vi "ErrorStructureDrawer-main.vi"(8 "Error In":errorcluster, 11 "VI reference":refnum<vi>) -> (0 "Error Out":errorcluster, 3 "VI reference (dup)":refnum<vi>)   [LabVIEW 2017, in "ErrorStructureDrawer.lvlib"]
doc: "Main VI for drawing an error structure around code using VI scripting."
uses:
  ErrorStructureDrawer.lvlib
panel:
  # "Copyright 2020, Stuart J. Box\n\nRedistribution and use in source and binary forms, with or without modification, are permitted provided that the following conditions are met:\n\n1. Redistributions of source code must retain the above copyright notice, this list of conditions and the following disclaimer.\n\n2. Redistributions in binary form must reproduce the above copyright notice, this list of conditions and the following disclaimer in the documentation and/or other materials provided with the distribution.\n\n3. Neither the name of the copyright holder nor the names of its contributors may be used to endorse or promote products derived from this software without specific prior written permission.\n\nTHIS SOFTWARE IS PROVIDED BY THE COPYRIGHT HOLDERS AND CONTRIBUTORS \"AS IS\" AND ANY EXPRESS OR IMPLIED WARRANTIES, INCLUDING, BUT NOT LIMITED TO, THE IMPLIED WARRANTIES OF MERCHANTABILITY AND FITNESS FOR A PARTICULAR PURPOSE ARE DISCLAIMED. IN NO EVENT SHALL THE COPYRIGHT HOLDER OR CONTRIBUTORS BE LIABLE FOR ANY DIRECT, INDIRECT, INCIDENTAL, SPECIAL, EXEMPLARY, OR CONSEQUENTIAL DAMAGES (INCLUDING, BUT NOT LIMITED TO, PROCUREMENT OF SUBSTITUTE GOODS OR SERVICES; LOSS OF USE, DATA, OR PROFITS; OR BUSINESS INTERRUPTION) HOWEVER CAUSED AND ON ANY THEORY OF LIABILITY, WHETHER IN CONTRACT, STRICT LIABILITY, OR TORT (INCLUDING NEGLIGENCE OR OTHERWISE) ARISING IN ANY WAY OUT OF THE USE OF THIS SOFTWARE, EVEN IF ADVISED OF THE POSSIBILITY OF SUCH DAMAGE."
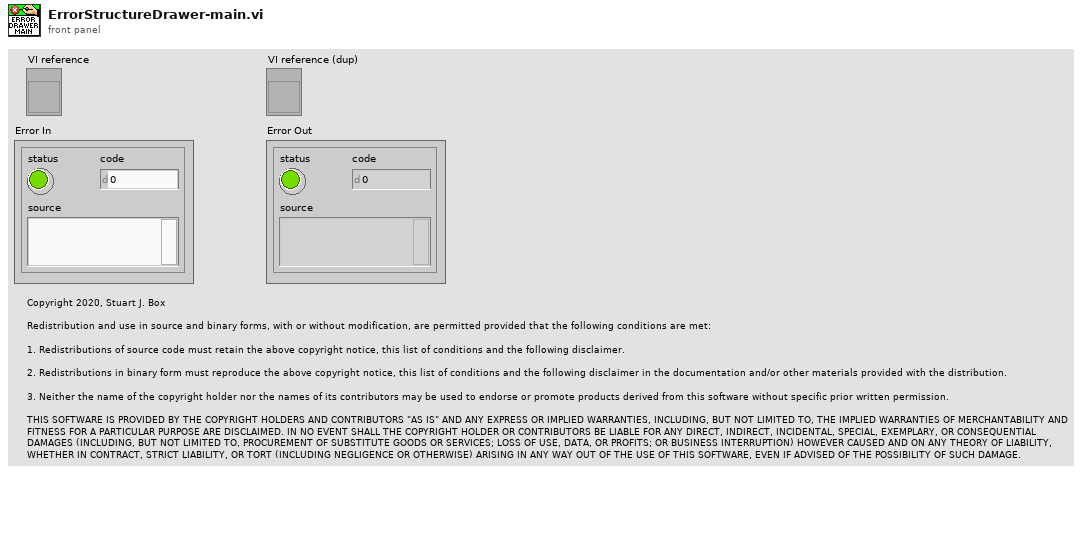
[diagram p1: front panel]
types:
  T1 = typedef "ErrorStructureDrawer.lvlib/ErrorTerminals.ctl" = cluster{"Control":refnum<vi>, "Indicator":refnum<vi>, "Control is new?":bool, "Indicator is new?":bool}
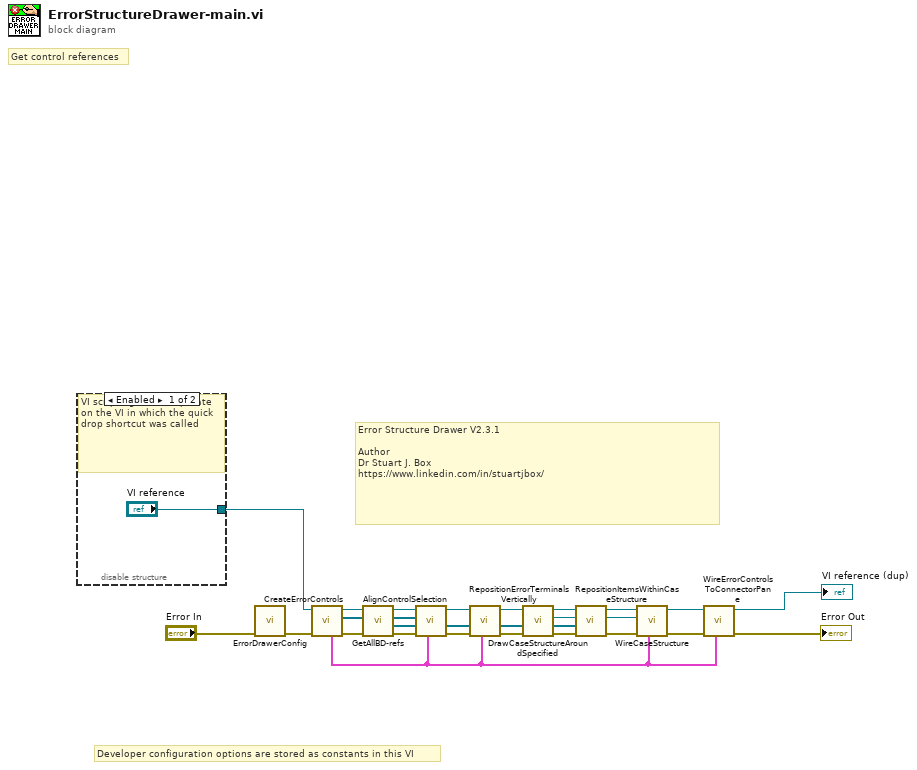
[diagram p0: block diagram]
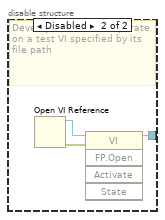
[diagram p2: hidden frame]
diagram:
  # "Error Structure Drawer V2.3.1\n\nAuthor\nDr Stuart J. Box\nhttps://www.linkedin.com/in/stuartjbox/"
  # "Developer configuration options are stored as constants in this VI"
  # "Get control references"
  n1 = disable-structure shown="Enabled" {
    disable-tunnel: ["VI reference" w31] -> w4
    frame Enabled {
      # "VI scripting mode - operate on the VI in which the quick drop shortcut was called"
    }
    frame Disabled {
      # "Development mode: operate on a test VI specified by its file path"
      n2 = Open VI Reference() -> (vi reference=w30:refnum<vi>, error out=w32:errorcluster)  [unwired: 6 in]
      n3 = invoke class="VI" method="FP.Open"(reference=w30, error in=w32) -> (reference out=w31:refnum<vi>)  [unwired: 3 in, 4 out]
    }
  }
  n4 = call "ErrorDrawerConfig.vi"("Error In"="Error In") -> ("Error Out"=w8:errorcluster)  [unwired: 10 in]
  n5 = call "CreateErrorControls.vi"("error in (no error)"=w8, "VI in"=w4) -> ("error out"=w12:errorcluster, "Control terminals on top-level"=w10:refnum<vi>[], "VI out (dup)"=w11:refnum<vi>, "Error terminals"=w1:T1)  [unwired: 6 in]
  n6 = call "GetAllBD-refs.vi"("error in (no error)"=w12, "Excluded objects"=w10, "VI ref in"=w11) -> ("error out"=w24:errorcluster, "All block diagram items (-filter)"=w21:refnum<vi>[], "Excluded objects out (dup)"=w23:refnum<vi>[], "VI ref out (dup)"=w22:refnum<vi>)  [unwired: 5 in]
  n7 = call "AlignControlSelection.vi"("Error terminals"=w1, "error in (no error)"=w24, "Item to enclose in case structure"=w21, "Control terminals on top-level"=w23, "VI in"=w22) -> ("error out"=w18:errorcluster, "Item to enclose in case structure (dup)"=w16:refnum<vi>[], "VI out (dup)"=w15:refnum<vi>)  [unwired: 4 in]
  n8 = call "RepositionErrorTerminalsVertically.vi"("Error terminals"=w1, "error in (no error)"=w18, "Item to enclose in case structure"=w16, "VI in"=w15) -> ("error out"=w9:errorcluster, "Item to enclose in case structure (dup)"=w17:refnum<vi>[], "VI out (dup)"=w14:refnum<vi>)  [unwired: 5 in]
  n9 = call "DrawCaseStructureAroundSpecified.vi"("error in (no error)"=w9, "Item to enclose in case structure"=w17, "VI ref in"=w14) -> ("error out"=w28:errorcluster, "Items inside case structure"=w25:refnum<vi>[], "New case structure"=w26:refnum<vi>, "VI ref out (dup)"=w27:refnum<vi>)  [unwired: 5 in]
  n10 = call "RepositionItemsWithinCaseStructure.vi"("error in (no error)"=w28, "Items inside case structure"=w25, "New case structure ref"=w26, "VI ref in"=w27) -> ("error out"=w20:errorcluster, "New case structure ref (dup)"=w19:refnum<vi>, "VI ref out (dup)"=w3:refnum<vi>)  [unwired: 5 in]
  n11 = call "WireCaseStructure.vi"("Error terminals"=w1, "error in (no error)"=w20, "New case structure ref"=w19, "VI ref in"=w3) -> ("error out"=w13:errorcluster, "VI ref out (dup)"=w2:refnum<vi>)  [unwired: 6 in]
  n12 = call "WireErrorControlsToConnectorPane.vi"("Error terminals"=w1, "error in (no error)"=w13, "VI"=w2) -> ("error out"=→"Error Out":errorcluster, "VI (dup)"=→"VI reference (dup)":refnum<vi>)  [unwired: 7 in]
